vi "Write Periodic Delay Parameters.vi"(10 "Periodic Delay Parameters":refnum<vi>, 11 "User Interface in":refnum<class "User Interface.lvclass">) -> (3 "User Interface out":refnum<class "User Interface.lvclass">)   [LabVIEW 2016, in "_User Interface.lvlib" / "User Interface.lvclass"]
uses:
  User Interface.lvclass
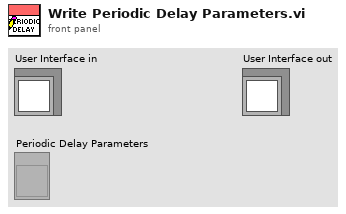
[diagram p1: front panel]
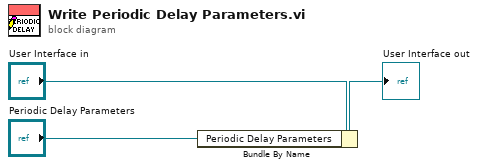
[diagram p0: block diagram]
diagram:
  n1 = Bundle By Name(cluster="User Interface in", "Periodic Delay Parameters"="Periodic Delay Parameters") -> (→"User Interface out":refnum<class "User Interface.lvclass">)
